vi "Arduino_Communication.vi"() -> ()   [LabVIEW 2022 SP3]
uses:
  2f7f86cf-63f6-4082-8031-e41d6b4aad7a.vi
  <vilib>/Instr/_visa.llb/VISA Configure Serial Port (Instr).vi
panel:
  in  "Read Position":bool
  out "Current Position":string
  in  "Serial":bool
  in  "Baud rate (9600)":u32=9600
  in  "VISA resource name":refnum<visa-resource-name>="COM9"
  in  "Forward":bool
  in  "Stop":bool
  in  "Back":bool
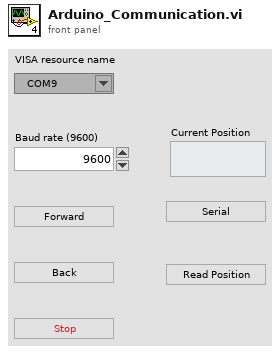
[diagram p1: front panel]
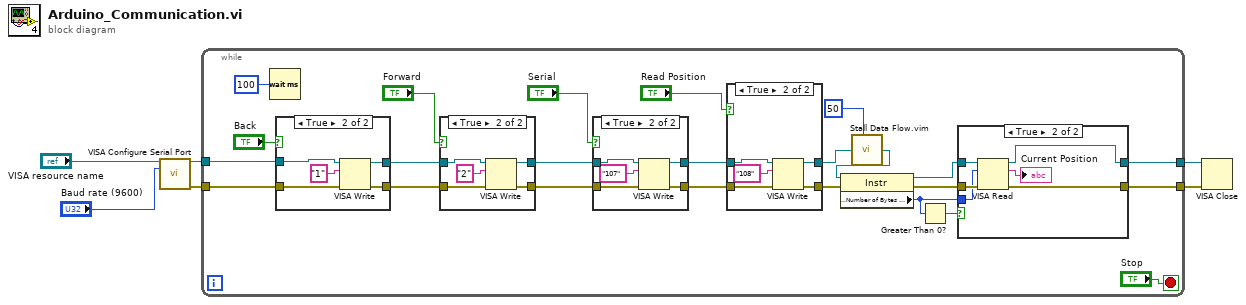
[diagram p0: block diagram]
diagram:
  n1 = call-poly "VISA Configure Serial Port"("VISA resource name"="VISA resource name", "baud rate (9600)"="Baud rate (9600)") -> ("VISA resource name out"=w6:refnum<visa-resource-name>, "error out"=w4:errorcluster)  [unwired: 12 in]
  n2 = while {
    tunnel: w6 -> [w30]
    tunnel: [w28] -> w5
    tunnel: w4 -> [w27]
    tunnel: [w25] -> w3
    stop <- "Stop" stop-if-true
    n3 = Wait (ms)(milliseconds to wait=u32 100) -> ()  [unwired: 1 out]
    n4 = case shown="True" "Back" {
      tunnel: w30 -> [w54 w59]
      tunnel: [w54 w58] -> w29
      tunnel: w27 -> [w53 w57]
      tunnel: [w53 w56] -> w26
      frame False {
      }
      frame True {
        n5 = VISA Write(VISA resource name=w59, write buffer="1", error in (no error)=w57) -> (VISA resource name out=w58:refnum<visa-resource-name>, error out=w56:errorcluster)  [unwired: 1 out]
      }
    }
    n6 = case shown="True" "Forward" {
      tunnel: w29 -> [w61 w66]
      tunnel: [w61 w65] -> w16
      tunnel: w26 -> [w60 w64]
      tunnel: [w60 w63] -> w15
      frame False {
      }
      frame True {
        n7 = VISA Write(VISA resource name=w66, write buffer="2", error in (no error)=w64) -> (VISA resource name out=w65:refnum<visa-resource-name>, error out=w63:errorcluster)  [unwired: 1 out]
      }
    }
    n8 = case shown="True" "Serial" {
      tunnel: w16 -> [w39 w44]
      tunnel: [w39 w43] -> w12
      tunnel: w15 -> [w38 w42]
      tunnel: [w38 w41] -> w11
      frame False {
      }
      frame True {
        n9 = VISA Write(VISA resource name=w44, write buffer="107", error in (no error)=w42) -> (VISA resource name out=w43:refnum<visa-resource-name>, error out=w41:errorcluster)  [unwired: 1 out]
      }
    }
    n10 = case shown="True" "Read Position" {
      tunnel: w12 -> [w32 w37]
      tunnel: [w32 w36] -> w9
      tunnel: w11 -> [w31 w35]
      tunnel: [w31 w34] -> w10
      frame False {
      }
      frame True {
        n11 = VISA Write(VISA resource name=w37, write buffer="108", error in (no error)=w35) -> (VISA resource name out=w36:refnum<visa-resource-name>, error out=w34:errorcluster)  [unwired: 1 out]
      }
    }
    n12 = call "Stall Data Flow.vim"("value in"=w9, "milliseconds to wait"=u32 50) -> ("value out"=w8:refnum<visa-resource-name>)  [unwired: 1 out]
    n13 = property class="Instr"(reference=w8, error in=w10) -> (reference out=w24:refnum<visa-resource-name>, error out=w23:errorcluster, "Serial Settings:Number of Bytes at Serial Port"=w21:u32)
    n14 = Greater Than 0?(x=w21) -> (x > 0?=w22:bool)
    n15 = case shown="True" w22 {
      tunnel: w24 -> [w46 w52]
      tunnel: [w46 w51] -> w28
      tunnel: w23 -> [w45 w50]
      tunnel: [w45 w49] -> w25
      tunnel: w21 -> [_ w48]
      frame False {
      }
      frame True {
        n16 = VISA Read(VISA resource name=w52, byte count=w48, error in (no error)=w50) -> (VISA resource name out=w51:refnum<visa-resource-name>, read buffer=→"Current Position":string, error out=w49:errorcluster)  [unwired: 1 out]
      }
    }
  }
  n17 = VISA Close(VISA resource name=w5, error in (no error)=w3) -> ()  [unwired: 1 out]
